vi "GetVersionSerializableData.vi"(10 "Version":u16, 11 "BlueSerializable in":refnum<class "BlueSerializable.lvclass">) -> (0 "error out":errorcluster, 1 "Found?":bool, 2 "SerializableData":variant, 3 "BlueSerializable out":refnum<class "BlueSerializable.lvclass">)   [LabVIEW 2019, in "BlueSerialization.lvlib" / "BlueSerializable.lvclass"]
uses:
  BlueSerializable.lvclass
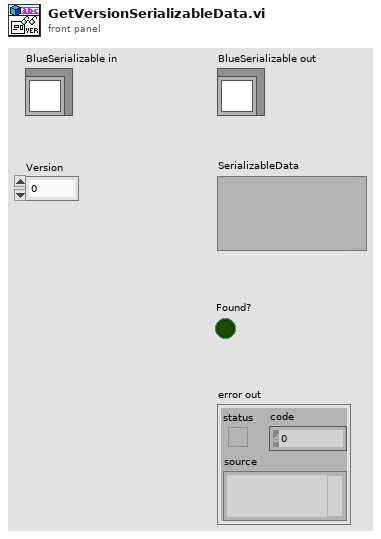
[diagram p1: front panel]
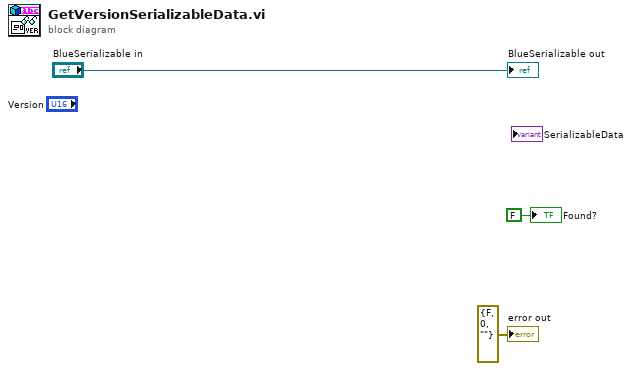
[diagram p0: block diagram]
diagram:
  "error out" <- errorcluster {"status"=FALSE, "code"=0, "source"=""} ("error out")
  "BlueSerializable out" <- "BlueSerializable in"
  "Found?" <- FALSE ("Found?")
